vi "Write_out_serial_log.vi"(0 "Header message":string) -> ()   [LabVIEW 2010]
uses:
  Serial_Logging_Global.vi
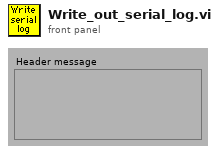
[diagram p1: front panel]
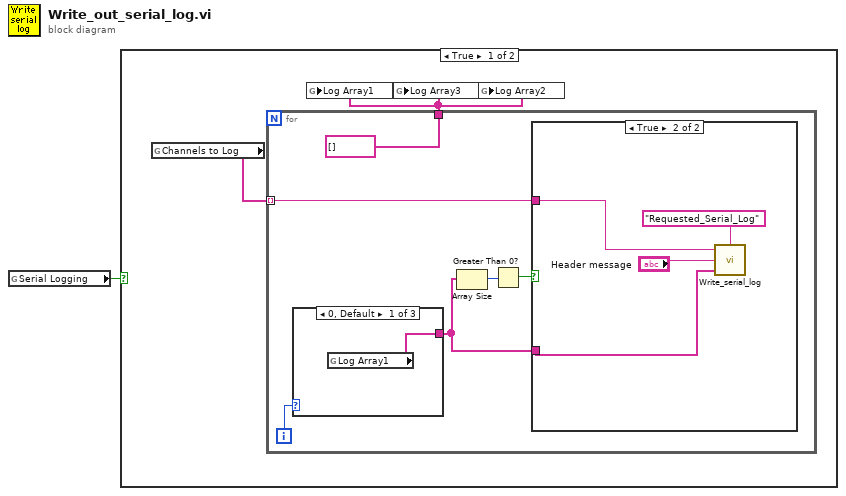
[diagram p0: block diagram]
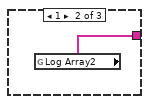
[diagram p3: hidden frame]
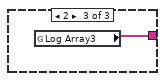
[diagram p4: hidden frame]
diagram:
  n1 = global read "Serial_Logging_Global.vi" "Serial Logging"() -> (w1:bool)
  n2 = case shown="True" w1 {
    frame True {
      n3 = global read "Serial_Logging_Global.vi" "Channels to Log"() -> (w3:string[])
      n4 = for {
        tunnel: w3 -> [w8] mode=indexing
        tunnel: [string[] [] ("Log Array1")] -> w2
        i -> [w9]
        n5 = case shown="0, Default" w9 {
          tunnel: [w14 w15 w16] -> w7
          frame 0, Default {
            n6 = global read "Serial_Logging_Global.vi" "Log Array1"() -> (w14:string[])
          }
          frame 1 {
            n7 = global read "Serial_Logging_Global.vi" "Log Array2"() -> (w15:string[])
          }
          frame 2 {
            n8 = global read "Serial_Logging_Global.vi" "Log Array3"() -> (w16:string[])
          }
        }
        n9 = Array Size(array=w7) -> (size(s)=w6:i32)
        n10 = Greater Than 0?(x=w6) -> (x > 0?=w5:bool)
        n11 = case shown="True" w5 {
          tunnel: w8 -> [_ w13]
          tunnel: w7 -> [_ w12]
          frame False {
          }
          frame True {
            n12 = call "Write_serial_log.vi"("Log Type"="Requested_Serial_Log", "Log Array"=w12, "Header message"="Header message", "Channel Name"=w13) -> ()  [unwired: 1 out]
          }
        }
      }
      n13 = global write "Serial_Logging_Global.vi" "Log Array1"(w2) -> ()
      n14 = global write "Serial_Logging_Global.vi" "Log Array3"(w2) -> ()
      n15 = global write "Serial_Logging_Global.vi" "Log Array2"(w2) -> ()
    }
    frame False {
    }
  }
